vi "Clean up JSON.vi"(8 "error in (no error)":errorcluster, 11 "Content JSON":string="```json\\n{\\n  \\\"Manufacturer\\\": \\\"JYSK\\\",\\n  \\\"Voltage\\\": 1.2,\\n  \\\"Capacity\\\": 2400,\\n  \\\"Error\\\": \\\"\\\"\\n}\\n```") -> (0 "error out":errorcluster, 3 "Cleaned up JSON":string)   [LabVIEW 2025]
doc: "Clean up the JSON received as a response content from the Open AI API"
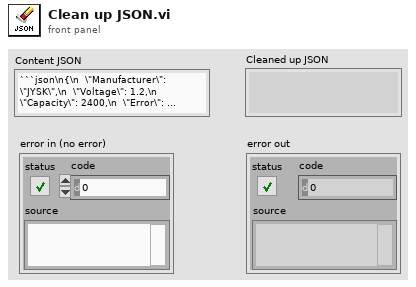
[diagram p1: front panel]
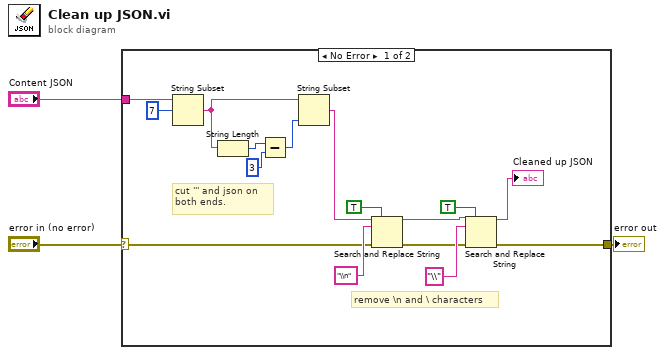
[diagram p0: block diagram]
diagram:
  n1 = case shown="No Error" "error in (no error)" {
    selector: "error in (no error)" -> [w5 w20]
    tunnel: "Content JSON" -> [w12 _]
    tunnel: [w4 w20] -> w1
    frame No Error {
      # "remove \\n and \\ characters"
      # "cut ''' and json on \nboth ends."
      n2 = String Subset(string=w12, offset (0)=7) -> (substring=w9:string)  [unwired: 1 in]
      n3 = String Length(string=w9) -> (length=w10:i32)
      n4 = Subtract(x=w10, y=3) -> (x-y=w8:i32)
      n5 = String Subset(string=w9, length (rest)=w8) -> (substring=w6:string)  [unwired: 1 in]
      n6 = Search and Replace String(replace all?=TRUE ("replace all? (F)"), input string=w6, search string="\\n", error in=w5) -> (result string=w15:string, error out=w14:errorcluster)  [unwired: 4 in, 2 out]
      n7 = Search and Replace String(replace all?=TRUE ("replace all? (F)"), input string=w15, search string="\\", error in=w14) -> (result string=→"Cleaned up JSON":string, error out=w4:errorcluster)  [unwired: 4 in, 2 out]
    }
    frame Error {
    }
  }
  "error out" <- w1
